vi "AlliGator Phasor Ratio Actions.vi"(0 "AlliGator Q Elements in":T6[](array[typedef]), 1 "VI in":refnum<vi>, 2 "Script in":bool, 5 "data value reference in":refnum<data-value>, 7 "AlliGator Q Event in":T7=enum."GUI:Idle", 9 "Data":variant, 11 "error in (no error)":errorcluster, 12 "AlliGator Ctrl Refnums":T8) -> (3 "Script out":bool, 4 "AlliGator Q Elements out":T6[](array[typedef]), 6 "Data Value Reference out":refnum<data-value>, 10 "[Notebook Message]":T1[](array[typedef]) {"Message Style"."Font Size" min=6.0 step=1.0}, 15 "error out":errorcluster)   [LabVIEW 2021, in "AlliGator Action Engine.lvlib"]
doc: "Processes AlliGator phasor ratio-related actions."
uses:
  AlliGator Action Engine.lvlib
  Internal Variables/AlliGator Internal Variables v2.ctl
  <vilib>/vision/Image Controls.llb/IMAQ Image.ctl
  Internal Variables/AlliGator Gate Image Set.ctl
  Files/AlliGator FLI Dataset Type.ctl
  Files/AlliGator Data Series Type.ctl
  Dual-Channel Datasets/AlliGator Dataset Channel.ctl
  Settings/AlliGator Gate Arithmetic.ctl
  Source Image/AlliGator Displayed Image.ctl
  Image/Named ROI Description.ctl
  Phasor Graph/AlliGator Decay Metadata v3.ctl
  Decay Analysis/Decay Preprocessing/AlliGator Decay Background Subtraction Info.ctl
  Decay Analysis/Decay Preprocessing/AlliGator Baseline Subtraction Method.ctl
  Graphs/XY Graph/XY Graph Plot Shift Parameters.ctl
  Graphs/XY Graph/XY Graph Plot Shift Method.ctl
  Decay Analysis/Decay Preprocessing/AlliGator Decay Extrapolation Parameters.ctl
  Phasor/Calibration Phasor (m, phi).ctl
  Phasor/Phasor Reference Series.ctl
  Phasor/Phasor Calibration Map v2.ctl
  Phasor/Phasor (g, s).ctl
  Phasor Graph/AlliGator Raw Phasor Plot Data v5.ctl
  Phasor/Phasor Standard Deviation Options.ctl
  Phasor Plot/AlliGator Phasor Multi-Harmonic Data.ctl
  Phasor/Phasor Harmonic Data.ctl
  Decay Fit Parameter Map/AlliGator Decay Fit Options & Parameters v3.ctl
  Fits/IRF(X)PSED/Decay Fit Options v3.ctl
  Fits/Decay Convolution/Decay Model.ctl
  Fits/Residual Type.ctl
  Fits/IRF(X)PSED/Fit Weights Type.ctl
  Fits/Non-linear Fitting Method v2.ctl
  Fits/Fit Calculation Method.ctl
  Fits/Non-linear Fitting Algorithm.ctl
  Decay Analysis/Decay Fit/AlliGator Decay Fit Parameter Constraints 2.ctl
  Fits/IRF(X)PSED/Decay Fit Parameters In List.ctl
  Fits/IRF(X)PSED/MLE Baseline Offset Type.ctl
  Decay Analysis/Decay Preprocessing/AlliGator Decay Preprocessing Parameters.ctl
  Fits/IRF(X)PSED/Decay Fit Parameters & Derived Quantities List v2.ctl
  Fits/IRF(X)PSED/Decay Fit Result Constraint.ctl
  Decay Fit Parameter Map/AlliGator Parameter Maps Data.ctl
  AlliGator Q Event.ctl
  GUI/AlliGator Ctrl Refnums.ctl
  GUI/AlliGator Other Ctrl Refnums.ctl
  GUI/AlliGator State Indicator.ctl
  GUI/AlliGator Main Window Tabs.ctl
  GUI/AlliGator Phasor Plot Ctrl Refnums.ctl
  GUI/AlliGator Phasor Graph Ctrl Refnums.ctl
  Phasor/Phasor Calibration Type.ctl
  GUI/AlliGator Dataset Ctrl Refnums.ctl
  GUI/AlliGator Registered Events Ctrl Refnums.ctl
  GUI/AlliGator Image Histogram Control Refnums.ctl
  Histograms/Linear Histogram Options.ctl
  Histograms/Histogram Bin Option.ctl
  Histograms/Histogram Bin Position.ctl
  Decay Fit Parameter Map/AlliGator Decay Fit Map Control Refnums.ctl
  Parameter Map/AlliGator Parameter Map Control Refnums.ctl
  AlliGator Q Element.ctl
  Notebook/Notebook Message Object.ctl
  Rich Text Box/Text Formatting.ctl
  Rich Text Box/Text Colors.ctl
  Rich Text Box/Text Style.ctl
  Rich Text Box/Text Alignment.ctl
  Rich Text Box/Text Format List.ctl
  Phasor Ratio/AlliGator Phasor Ratio at Mouse Location Data.ctl
  Graphs/XY Graph/XY Graph Mouse Click Event Data.ctl
  Graphs/XY Graph/XY Graph Refnum.ctl
  <vilib>/Utility/miscctls.llb/LVPoint32TypeDef.ctl
  Phasor Ratio/AlliGator Phasor Reference Data.ctl
  Alligator Elements Order in Action Stack.ctl
  AlliGator State Indicators List.ctl
  Globals, Variables, Constants/AlliGator Variables List.ctl
  Variant/Variant to Data/Variant to I32.vi
  Graphs/Get Plot at Mouse Click (XY Graph)/Get Plot at Mouse Click [AAC].vi
  Variant/Variant to Data/Variant to Boolean.vi
  Variant/Variant to Data/Variant to Path.vi
  AlliGator Add Single Action to Stack.vi
  Variant/Variant to Data/Variant to DBL.vi
  Variant/Variant to Data/Variant to Data.lvlib
  GUI/GUI.lvlib
  Source Image/AlliGator Source Image.lvlib
  Phasor Graph/AlliGator Phasor Graph.lvlib
  Phasor Ratio/AlliGator Phasor Ratio.lvlib
  Internal Variables/AlliGator Internal Variables.lvlib
  Graphs/XY Graph/XY Graph Add-Ons.lvlib
  Graphs/Graphs.lvlib
  Globals, Variables, Constants/AlliGator Globals, Variables & Constants.lvlib
  GUI/AlliGator GUI.lvlib
  Settings/AlliGator Settings.lvlib
  Phasor Calibration/AlliGator Phasor Calibration.lvlib
  Notebook/Notebook.lvlib
  Phasor/Phasor.lvlib
  Image/Image.lvlib
  Decay Analysis/Decay Preprocessing/AlliGator Decay Preprocessing.lvlib
  Files/AlliGator Files.lvlib
  Phasor Plot/AlliGator Phasor Plot.lvlib
  Fits/Fits.lvlib
  Decay Analysis/Decay Fit/AlliGator Decay Fit.lvlib
  Decay Fit Parameter Map/AlliGator Decay Fit Parameter Map.lvlib
  Rich Text Box/Rich Text Box.lvlib
  Dual-Channel Datasets/AlliGator Dual-Channel Datasets.lvlib
  Histograms/Histogram Window.lvlib
  Parameter Map/AlliGator Parameter Map.lvlib
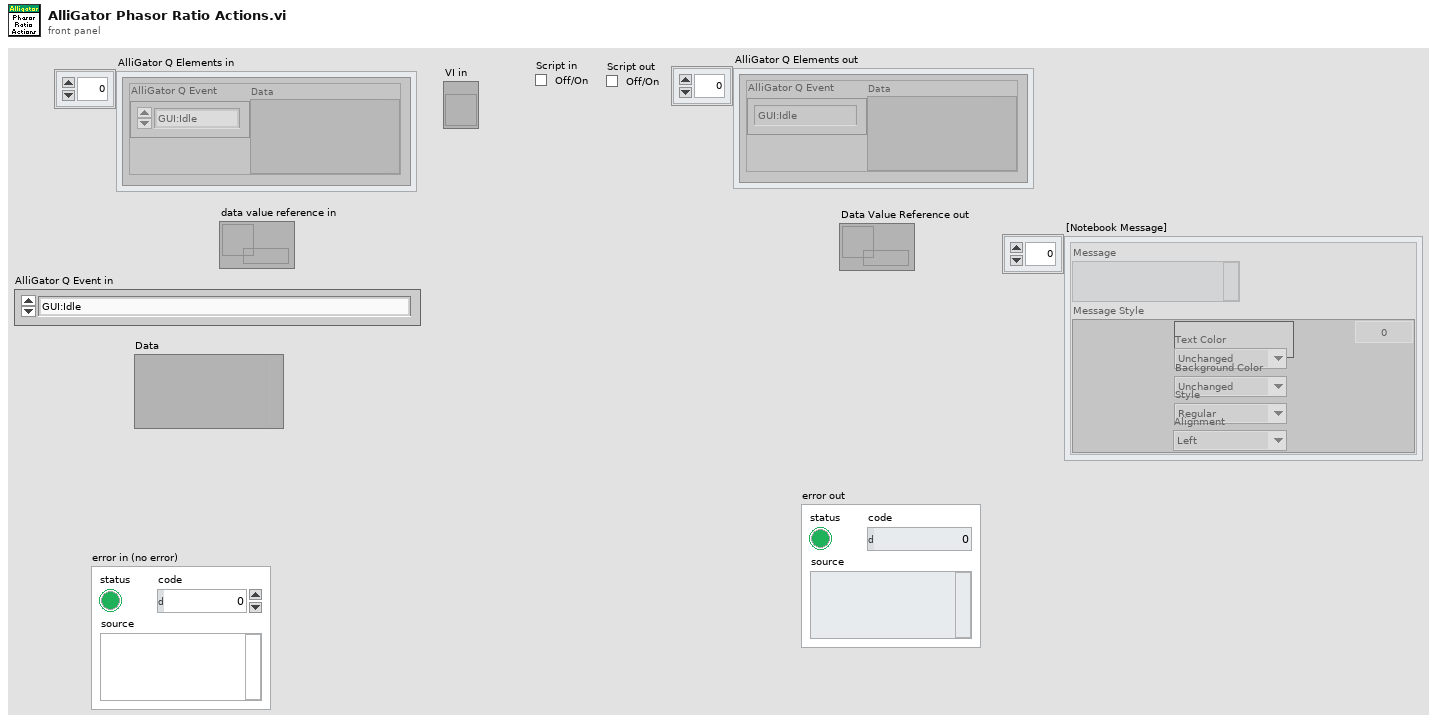
[diagram p1: front panel]
types:
  T1 = typedef "Notebook.lvlib/Notebook Message Object.ctl" = cluster{"Message":string, "Message Style":T2}
  T2 = typedef "Rich Text Box.lvlib/Text Formatting.ctl" = cluster{"Font":string, "Text Color":T3, "Background Color":T3, "Style":T4, "Font Size":dbl, "Alignment":T5}
  T3 = typedef "Rich Text Box.lvlib/Text Colors.ctl" = enum16{"Unchanged", "Black", "Blue", "Cyan", "Maroon", "Gray", "Violet", "Green", "Light Green", "Orange", "Yellow", "Magenta", "Red", "White"}
  T4 = typedef "Rich Text Box.lvlib/Text Style.ctl" = enum16{"Regular", "Bold", "Italic", "Underline", "Strikeout"}
  T5 = typedef "Rich Text Box.lvlib/Text Alignment.ctl" = enum16{"Left", "Right", "Center"}
  T6 = typedef "AlliGator Action Engine.lvlib/AlliGator Q Element.ctl" = cluster{"AlliGator Q Event":T7, "Data":variant}
  T7 = typedef "AlliGator Action Engine.lvlib/AlliGator Q Event.ctl" = enum16{"---- Files ----", "Files:Set Batch Export Files To Save", "Files:Set Dataset Loading & Pre-processing Options", "Files:Check #Frames in Dataset", "Files:Increment Frame Index", "Files:Open Mask Image", "Files:Open White Light Image", "Files:Open Single Dataset", "Files:New Folder of Folders Selected", "Files:Load File (all Types)_Scriptable", "Files:Move Flattened Series to Folders Series", "Files:Select Folder", "Files:Load FLI Dataset", "Files:Load Swiss SPAD 1 Dataset", "Files:Load Swiss SPAD 2 Dataset", "Files:Load .sdt FLI Dataset", "Files:Load .ptu FLI Dataset", "Files:Load .bin FLI Dataset", "Files:Load Single Gate Image Folder", "Files:Load I/m/phi Dataset (deprecated)", "Files:Load Single Image", "Files:Subtract Background File", "Files:Export FLI Dataset", "Files:Load HDF5 FLI Dataset", "Files:Set Destination File Path", "Files:Save Mask Image", "Files:Batch Conversion", "Files:New Folder Selected", "Files:Close FLI Dataset", "Files:Close FLI Dataset Series", "Files:Close White Light Image", "Files:Close Mask Image", "---- FLI Dataset ----", "FLI Dataset:Channel Arithmetic", "FLI Dataset:Export Average Lifetime Map as ASCII", "FLI Dataset:Export User-Defined Quantity Map as ASCII", "FLI Dataset:Python Function FLI Dataset Event", "FLI Dataset:ROI Analysis", "FLI Dataset:Tilted Logistic Square Gated IRF Characteristics Map", "FLI Dataset:Logistic Square Gated IRF Characteristics Map", "FLI Dataset:Square Gated IRF Characteristics Map", "FLI Dataset:Multi-ROI Single-Pixel Phasor Analysis", "FLI Dataset:Multi-ROI Single-Pixel NLSF Analysis", "FLI Dataset:All ROIs IRF Extraction", "FLI Dataset:All ROIs Decay Fit Non-Interactive (Fast + Individual IRF)", "FLI Dataset:All ROIs Phasor Analysis", "FLI Dataset:All ROIs Decay Fit", "FLI Dataset:Fluorescence Decay Statistics", "FLI Dataset:Update Decay Statistics Graph", "FLI Dataset:Get Decay from ROI", "FLI Dataset:All ROIs Average Lifetimes", "FLI Dataset:Save/Load Local IRFs", "FLI Dataset:Clear Local IRFs", "FLI Dataset:Phasor Calibration Maps (# Gates Series) Script", "FLI Dataset:Calibrated Phasor Map Series", "---- FLI Dataset Series ----", "FLI Dataset Series:Sum All Datasets in Series", "FLI Dataset Series:Add Dataset to Accumulated Dataset", "FLI Dataset Series:Display Accumulated Dataset", "FLI Dataset Series:Clear Dataset Series Sum", "FLI Dataset Series:Time-Series Analysis (NLSF)", "FLI Dataset Series:Time-Series Analysis (Phasor)", "---- Image ----", "Image:Update Image Profile Plots", "Image:Image Histogram Cursor Move", "Image:Image Histogram", "Image:Image Contrast", "Image:Set Image Histogram Cursor Move Flag", "Image:Clear Image Overlay", "Image:Use ROI as Search Area", "Image:Set ROI Diameter", "Image:Save Image Data as TIFF", "Image:Save Displayed Image with Overlay", "Image:Save Image Overlay Only", "Image:Save Image as Hot Pixel Mask", "Image:Change Source Image Color Palette", "Image:Copy Image to Clipboard", "Image:Source Image ROI Selection", "Image:Delete All ROIs", "Image:Delete All Unselected ROIs", "Image:Delete ROI", "Image:Merge All ROIs", "Image:Store ROI", "Image:Source Image ROI Storage", "Image:Export ROI Description to Notebook", "Image:Save ROI", "Image:Load ROI", "Image:Paste ROI Definition", "Image:Clear ROI", "Image:Identify ROIs in Mask Image", "Image:Create Complementary ROI", "Image:Create Contour ROI", "Image:Create ROI(s) from Pixels with Peak above Min_Scriptable", "Image:Create ROI(s) from Pixels with Intensity above Min_Scriptable", "Image:Compute ROI Statistics", "Image:Delete ROI(s) based on ROI Characteristics", "Image:Create ROI Grid", "Image:ROI to Individual Pixel ROIs", "Image:Python Function Source Image Event", "Image:Show Phasor Calibration Map ROI Centers", "Image:Convert ROI to Mask Image", "Image:Mouse Move", "Image:Mouse Up", "Image:Set Source Image Mouse Move Flag", "Image:Add Scale Bar Overlay", "Image:Delete Existing ROIs Option", "Image:Overlay ROI Median", "Image:Check Current ROI", "Image:Update True Pixel Value", "---- Decay ----", "Decay:Clear IRF/Reference Plot", "Decay:Add Decay to Graph", "Decay:Smoothen Plot", "Decay:Smoothen Plot Tail", "Decay:Average Selected Plots", "Decay:Extract IRF", "Decay:Optimal IRF Extraction", "Decay:Threshold IRF", "Decay:Fit to Model IRF", "Decay:Fit IRF to Square Gate", "Decay:Fit IRF to Logistic Square Gate", "Decay:Fit IRF to Tilted Logistic Square Gate", "Decay:Create Bounding Cursors Set", "Decay:Export Bounding Cursors Definition to Notebook", "Decay:Denoise Plot", "Decay:Compute Cumulative Function", "Decay:Use as Reference Decay", "Decay:Show Reference Decay/IRF", "Decay:Extrapolate Decay", "Decay:Create Head & Tail Bounding Cursors", "Decay:Store Cursor-defined Head & Tail Fractions", "Decay:Rebin Plot", "Decay:1-Normalize Decay", "Decay:[0-1]-Normalize Plot", "Decay:Straighten Decay", "Decay:Shift Decay", "Decay:Fold Decay", "Decay:Fit Decay", "Decay:Global Fit of Selected Decays", "Decay:Post Global Fit Script", "Decay:Add Global Fit Parameters to Graph", "Decay:Add Decay Parameter(s) to Plot (Graph)", "Decay:Export Decay to Phasor Graph", "Decay:Compute Average Lifetime", "Decay:Plot Convolution", "Decay:Graph Tip Strip Update", "---- Decay Statistics ----", "Decay Statistics:Tip Strip Update", "---- Intensity Time Trace ----", "Intensity Time Trace:Use File Timestamp", "Intensity Time Trace:Load Intensity Corrections File", "Intensity Time Trace:Clear Intensity Corrections File", "Intensity Time Trace:Tip Strip Update", "---- Phasor Plot ----", "Phasor Plot:Build Phasor Plot", "Phasor Plot:Change Phasor Plot Color Palette", "Phasor Plot:Adjust Phasor Plot Display Range", "Phasor Plot:Highlight Image ROI in Phasor Plot", "Phasor Plot:Save Phasor Plot Image with Overlay", "Phasor Plot:Export Complex Phasor Map", "Phasor Plot:Export Phasor Ratio Map", "Phasor Plot:Export Average Lifetime Map", "Phasor Plot:Compute Phase Lifetime Histogram", "Phasor Plot:Compute Phasor Ratio Histogram", "Phasor Plot:Compute Phase Lifetime vs Intensity Scatter Plot", "Phasor Plot:Weber 2-Component Decomposition", "Phasor Plot:Update Phasor Color Map Vertices", "Phasor Plot:Clear Phasor Overlay", "Phasor Plot:Use Segment Extremities as References", "Phasor Plot:Use UC/Segment Intersections as References", "Phasor Plot:Use UC/Principal Axis Intersections as References", "Phasor Plot:Use UC/Linear Fit Intersections as References", "Phasor Plot:Update Phasor Plot Reference", "Phasor Plot:Show Local Phasor Info in Phasor Plot", "Phasor Plot:Update Phasor Plot State", "Phasor Plot:Phasor Plot ROI Storage", "Phasor Plot:Phasor Plot ROI Selection", "Phasor Plot:Python Function Phasor Plot Event", "Phasor Plot:Overlay Phasor ROI, Ratio or Map in Source Image", "Phasor Plot:Compute Decay of Selected Phasors", "Phasor Plot:Phasor at Image Pixel", "Phasor Plot:Mouse Move", "Phasor Plot:Mouse Up", "Phasor Plot:Display Range Mouse Move", "Phasor Plot:Set Mouse Move Flag", "Phasor Plot:Update True Phasor Plot Value", "---- Phasor Graph ----", "Phasor Graph:Get Phasor Value", "Phasor Graph:Create New Phasor Plot Dialog", "Phasor Graph:Update Last Phasor Value", "Phasor Graph:Update Phasor (m, phi)", "Phasor Graph:Remove Single Phasor from Plot", "Phasor Graph:Add Single Phasor to Plot", "Phasor Graph:Remove Phasor Plot", "Phasor Graph:Remove Selected Phasor Plots", "Phasor Graph:Clear Phasor Data", "Phasor Graph:Clear Phasor Graph", "Phasor Graph:Cursor Move", "Phasor Graph:Draw Cursor Connecting Line", "Phasor Graph:Clear Cursor Connecting Line", "Phasor Graph:Find UC Intersection", "Phasor Graph:Use UC/Cursor-Defined Line Intersections", "Phasor Graph:Use Selected Plots Fitted Line/UC Intersections", "Phasor Graph:Use Selected Plots Principal Axis/UC Intersections", "Phasor Graph:Show Single Phasor", "Phasor Graph:Save Single Phasor Plot", "Phasor Graph:Save All Phasor Plots", "Phasor Graph:Load Phasor Plot(s)", "Phasor Graph:Phasor Multiplication", "Phasor Graph:Compute Average Phasor", "Phasor Graph:Compute Multiple Average Phasors (Selected Plots)", "Phasor Graph:Export Single Phasor Plot Phase Lifetimes", "Phasor Graph:Parameter 2 vs Parameter 1 Scatter Plot", "Phasor Graph:Use Cursor n Location", "Phasor Graph:Set Reference n to Current Phase Lifetime Value", "Phasor Graph:Set Reference n to Lifetime Value", "Phasor Graph:Set Cursor n Location", "Phasor Graph:Save Phasor Graph Image", "Phasor Graph:Update SEPL Plot", "Phasor Graph:Export Single Phasor Plot Data", "Phasor Graph:Export Selected Phasor Plots Data", "Phasor Graph:Python Function Phasor Graph Event", "Phasor Graph:Tip Strip Update", "---- Calibration ----", "Calibration:Set Calibration Type", "Calibration:Load/Save Phasor Calibration", "Calibration:Load/Save Phasor Calibration Series", "Calibration:Load/Save Phasor Calibration Map", "Calibration:Use as Calibration", "Calibration:Compute Optimal Calibration from Phasor References", "Calibration:Clear Phasor Calibration", "Calibration:Single Phasor Calibration Information", "Calibration:Use as Calibration Series", "Calibration:Use as Calibration Map", "Calibration:Clear Calibration Series", "Calibration:Phasor Calibration Series Information", "Calibration:Clear Calibration Map", "Calibration:Phasor Calibration Map Information", "Calibration:Apply Phasor Calibration", "Calibration:Update Single Plot Calibration", "Calibration:Update Multiple Plots Calibration", "Calibration:Clear Single Plot Calibration", "Calibration:Clear All Plots Calibrations", "Calibration:Clear Plot(s) Calibration(s)?", "---- Phasor Ratio ----", "Phasor Ratio:Clear Reference n", "Phasor Ratio:Toggle Selected Plot(s)  Lock to Reference 1", "Phasor Ratio:Use as Reference n", "Phasor Ratio:Send Reference n to Notebook", "Phasor Ratio:Toggle Selected Plot(s)  Lock to Reference 2", "Phasor Ratio:Compute Phasor Ratio at Mouse Location", "Phasor Ratio:Compute Phasor Plot's Average Phasor Ratio", "Phasor Ratio:Compute Time-Series Phasor Ratios", "Phasor Ratio:Fit Line to Phasor Ratio Plot", "Phasor Ratio:Save References", "Phasor Ratio:Load References", "Phasor Ratio:Update Phasor Reference 1", "Phasor Ratio:Update Phasor Reference 2", "Phasor Ratio:Move Cursor n to Reference n", "Phasor Ratio:Use as Phasor Reference 1 Lifetime", "Phasor Ratio:Use as Phasor Reference 2 Lifetime", "Phasor Ratio:Export Phasor Ratio Map as ASCII", "Phasor Ratio:Tip Strip Update", "---- Lifetime & Other Parameters Graph ----", "Lifetime:Compute Sliced Mean, SDV and CV Plots", "Lifetime:Plot Decay Shifts", "Lifetime:Plot Histogram", "---- Decay Fit Parameter Map ----", "Decay Fit Parameter Map:Export ROI NLSF Data as ASCII", "Decay Fit Parameter Map:Set Decay Fit Parameter Map Selection", "Decay Fit Parameter Map:Build Decay Fit Parameter Map", "Decay Fit Parameter Map:Change Decay Fit Parameter Map Color Palette", "Decay Fit Parameter Map:Export Decay Fit Parameter Map Data as ASCII", "Decay Fit Parameter Map:Export All Decay Fit Parameter Maps Data as ASCII", "Decay Fit Parameter Map:Selected Parameter Scatterplot", "Decay Fit Parameter Map:Parameter 2 vs Parameter 1 Scatterplot", "Decay Fit Parameter Map:Save Decay Fit Parameter Map Image", "Decay Fit Parameter Map:Save-Load IRFs & Fit Data", "Decay Fit Parameter Map:Update Local Decay Plots", "Decay Fit Parameter Map:Python Function Decay Fit Parameters Map Event", "Decay Fit Parameter Map:Overlay Decay Fit Parameter Map in Source Image", "Decay Fit Parameter Map:Selected Parameter vs Intensity Scatterplot", "Decay Fit Parameter Map:Mouse Up", "Decay Fit Parameter Map:Mouse Move", "Decay Fit Parameter Map:Display Range Mouse Move", "Decay Fit Parameter Map:Change Map Resolution", "Decay Fit Parameter Map:Variance Significance Maps", "Decay Fit Parameter Map:Fit Result Constraints Window", "---- Parameter Map ----", "Parameter Map:Export ROI Parameters Data as ASCII", "Parameter Map:Delete Parameter Map Set", "Parameter Map:Update Parameter List", "Parameter Map:Build Parameter Map", "Parameter Map:Change Parameter Map Color Palette", "Parameter Map:Export Parameter Map Data as ASCII", "Parameter Map:Export All Parameter Maps Data as ASCII", "Parameter Map:Selected Parameter Scatterplot", "Parameter Map:Parameter 2 vs Parameter 1 Scatterplot", "Parameter Map:Selected Parameter vs Intensity Scatterplot", "Parameter Map:Save Parameter Map Image", "Parameter Map:Save-Load IRFs & Parameter Maps (TODO)", "Parameter Map:Set Parameter Map Selection", "Parameter Map:Python Function Parameter Map Event", "Parameter Map:Overlay Parameter Map in Source Image", "Parameter Map:Update Local Decay Plots", "Parameter Map:Mouse Up", "Parameter Map:Mouse Move", "Parameter Map:Display Range Mouse Move", "---- Generic Graph ----", "Generic Graph:Generic XY Graph Event", "Generic Graph:Python Function XY Graph Event", "Generic Graph:New Plot", "Generic Graph:Save Plot", "Generic Graph:XY Plot Histogram", "Generic Graph:Set XY Graph Plot Name", "Generic Graph:Set Last Cursor Style", "Generic Graph:Tip Strip Update", "---- GUI ----", "GUI:Start Script", "GUI:Type of Displayed Image Changed", "GUI:Gate Image Slide Changed", "GUI:Show Busy Icon", "GUI:Show Busy Icon & Abort Button", "GUI:Hide Busy Icon", "GUI:Hide Busy Icon & Abort Button", "GUI:Abort", "GUI:End Script", "GUI:Start Timing", "GUI:End Timing", "GUI:Set State Indicator", "GUI:Send Parameters JSON Strings to Clipboard", "GUI:Set Gate Step", "GUI:Idle", "GUI:Initialization", "GUI:Quit", "GUI:Increment Dataset Index", "GUI:Set Dataset Index to -1", "GUI:Time Series Slider Moved", "GUI:Time Series Slider Changed", "GUI:Toggle Playback or Loop", "GUI:Playback Script", "GUI:Set Phasor Frequency", "GUI:Open Window", "GUI:Start Test Script", "GUI:End Test Script", "DEBUG"}
  T8 = typedef "AlliGator GUI.lvlib/AlliGator Ctrl Refnums.ctl" = cluster{"Other AlliGator Ctrl Refnums":T9, "Phasor Plot Ctrl Refnums":T10, "Phasor Graph Ctrl Refnums":T11, "Dataset Control Refnums":T12, "Registered Events Ctrl Refnums":T13, "Image Histogram Ctrl Refnums":T14, "Decay Fit Map Ctrl Refnums":T15, "Parameter Map Ctrl Refnums":T16}
  T9 = typedef "AlliGator GUI.lvlib/AlliGator Other Ctrl Refnums.ctl" = cluster{"State Indicators":refnum<vi>, " Progress Bar":refnum<vi>, "Decay Graph Active":refnum<vi>, "Decay Statistics Bin":refnum<vi>, "Time Step":refnum<vi>, "Use File Timestamp":refnum<vi>, "Tab Control":refnum<vi>, "CPU":refnum<vi>, "Abort Fit":refnum<vi>, "Dataset File/Folder Path":refnum<vi>, "Abort ROI Creation":refnum<vi>, "Event LED":refnum<vi>, "Dataset File/Folder Path 2":refnum<vi>, "Dataset File/Folder Path 3":refnum<vi>, "Dataset File/Folder Path 4":refnum<vi>, "Dataset File/Folder Path 5":refnum<vi>, "Dataset File/Folder Path 6":refnum<vi>, "Dataset File/Folder Path 7":refnum<vi>, "Dataset File/Folder Path 8":refnum<vi>, "Dataset File/Folder Path 9":refnum<vi>, "Dataset File/Folder Path 10":refnum<vi>, "Dataset File/Folder Path 11":refnum<vi>}
  T10 = typedef "AlliGator GUI.lvlib/AlliGator Phasor Plot Ctrl Refnums.ctl" = cluster{"Phasor Ratio":refnum<vi>, "Modulus Lifetime":refnum<vi>, "Phasor at cursor (m, phi)":refnum<vi>, "Phase Lifetime":refnum<vi>, "Phasor at cursor (g, s)":refnum<vi>, "Phasor Plor Average Lifetime":refnum<vi>, "Phasor Plot Active":refnum<vi>, "Save Phasor Plot":refnum<vi>, "Image Overlay Color":refnum<vi>, "Phasor Plot Color Scale":refnum<vi>, "Reference 1 Button":refnum<vi>, "Reference 2 Button":refnum<vi>, "True Phasor Plot Value":refnum<vi>}
  T11 = typedef "AlliGator GUI.lvlib/AlliGator Phasor Graph Ctrl Refnums.ctl" = cluster{"Phasor Ratio":refnum<vi>, "Modulus Lifetime":refnum<vi>, "Phasor at cursor (m, phi)":refnum<vi>, "Phase Lifetime":refnum<vi>, "Phasor at cursor (g, s)":refnum<vi>, "Phasor Graph Average Lifetime":refnum<vi>, "Phasor Graph Active":refnum<vi>, "Save Phasor Graph":refnum<vi>, "Phasor Frame Slide":refnum<vi>, "Single Step Phasor":refnum<vi>, "Calibration Type":refnum<vi>, "Show Line":refnum<vi>, "Phase Lifetime 1":refnum<vi>, "Phase Lifetime 2":refnum<vi>, "Phasor Graph Frequency":refnum<vi>, "Phasor Reference 1 Control":refnum<vi>, "Phasor Reference 2 Control":refnum<vi>, "Calibration Lifetime":refnum<vi>, "Phase Lifetime SDV":refnum<vi>, "Average Lifetime SDV":refnum<vi>, "Phasor Ratio SDV":refnum<vi>, "Modulus Lifetime SDV":refnum<vi>}
  T12 = typedef "AlliGator GUI.lvlib/AlliGator Dataset Ctrl Refnums.ctl" = cluster{"Current Data":refnum<vi>, "Gate Image Slide":refnum<vi>, "Time Point Slide":refnum<vi>, "Current Time Stamp":refnum<vi>, "Save Image":refnum<vi>, "Displayed Image":refnum<vi>, "Overlay Mode":refnum<vi>, "Phasor Overlay Color":refnum<vi>, "Image Color Scale":refnum<vi>, "Use ROI as Search Area":refnum<vi>, "Source Image ROI Color":refnum<vi>, "True Pixel Value":refnum<vi>}
  T13 = typedef "AlliGator GUI.lvlib/AlliGator Registered Events Ctrl Refnums.ctl" = cluster{"Time Point Slider":refnum<vi>, "Phasor Plot Display Range":refnum<vi>, "Decay Graph":refnum<vi>, "Decay Statistics Graph":refnum<vi>, "Intensity Time Trace":refnum<vi>, "Phasor Graph":refnum<vi>, "Phasor Ratio Graph":refnum<vi>, "Lifetime Graph":refnum<vi>, "Phasor Plot Display":refnum<vi>, "Source Image Display":refnum<vi>, "Decay Fit Parameter Map Display Range":refnum<vi>, "Decay Fit Parameter Map Display":refnum<vi>, "Parameter Map Display Range":refnum<vi>, "Parameter Map Display":refnum<vi>, "Phasor Plot Display Range":refnum<vi>}
  T14 = typedef "AlliGator GUI.lvlib/AlliGator Image Histogram Control Refnums.ctl" = cluster{"Image Histogram":refnum<vi>, "Image Histogram Options":refnum<vi>, "Image Histogram Active":refnum<vi>, "Image Histogram Upper Percentile":refnum<vi>, "Image Histogram Lower Percentile":refnum<vi>, "Auto-Adjust Contrast":refnum<vi>}
  T15 = typedef "AlliGator Decay Fit Parameter Map.lvlib/AlliGator Decay Fit Map Control Refnums.ctl" = cluster{"Decay Fit Parameter Map Color Scale":refnum<vi>, "Decay Fit Parameter":refnum<vi>, "Max Parameter":refnum<vi>, "Min Parameter":refnum<vi>, "Decay Fit Parameter Map Display":refnum<vi>, "Decay Fit Parameter Map Display Range":refnum<vi>, "Decay Parameter Map X":refnum<vi>, "Decay Parameter Map Y":refnum<vi>, "Decay Parameter Map Value":refnum<vi>}
  T16 = typedef "AlliGator Parameter Map.lvlib/AlliGator Parameter Map Control Refnums.ctl" = cluster{"Parameter Map Color Scale":refnum<vi>, "Map Parameter":refnum<vi>, "Max Parameter":refnum<vi>, "Min Parameter":refnum<vi>, "Parameter Map Display":refnum<vi>, "Parameter Map Display Range":refnum<vi>, "Parameter Map Set":refnum<vi>, "Parameter Map X":refnum<vi>, "Parameter Map Y":refnum<vi>, "Parameter Map Value":refnum<vi>}
  T17 = typedef "Notebook.lvlib/Text Format List.ctl" = enum16{"Message", "Result", "Error", "Setting", "Verbose", "Warning"}
  T18 = typedef "AlliGator Phasor Ratio.lvlib/AlliGator Phasor Ratio at Mouse Location Data.ctl" = cluster{"Mouse Click Event Data":T19, "Interactive?":bool}
  T19 = typedef "XY Graph Add-Ons.lvlib/XY Graph Mouse Click Event Data.ctl" = cluster{"Multiplot XY Graph":T20, "Mouse Coordinates":T21}
  T20 = typedef "XY Graph Add-Ons.lvlib/XY Graph Refnum.ctl" = refnum<vi>
  T21 = typedef "LVPoint32TypeDef.ctl" = cluster{"Horizontal":i32, "Vertical":i32}
  T22 = typedef "AlliGator Phasor Ratio.lvlib/AlliGator Phasor Reference Data.ctl" = cluster{"Data Type":string, "Data":variant}
  T23 = typedef "AlliGator Action Engine.lvlib/Alligator Elements Order in Action Stack.ctl" = enum16{"Enqueue 2 AFTER 1", "Enqueue 2 BEFORE 1"}
  T24 = typedef "AlliGator Globals, Variables & Constants.lvlib/AlliGator Variables List.ctl" = enum16{"---- GUI ----", "GUI:Initialization Status", "GUI:State Indicators Refnum", "GUI:Original AlliGator Menu Items", "GUI:Current Action Loop State", "GUI:Script in progress", "GUI:Playback", "GUI:Loop Playback", "GUI:Search ROI Used", "GUI:Search ROI", "Decay Graph Max Legend Size", "Intensity Graph Max Legend Size", "Decay Statistics Graph Max Legend Size", "Phasor Graph Max Legend Size", "Phasor Ratio Graph Max Legend Size", "Lifetime Graph Max Legend Size", "---- Files ----", "Files:Export Dataset Frames as Individual Files", "Files:Show Batch Export Help Balloons", "Files:Frames in Dataset", "Files:ptu File Frame Start Indices", "Files:Current Frame in Dataset", "Files:Current Frame Timestamp", "Files:Dataset Loaded", "Files:Dataset Metadata", "Files:Dataset Channel", "Files:Dataset Data Description", "Files:Background Dataset Metadata", "Files:Background Dataset Channel", "Files:Background Dataset Data Description", "Files:Background File Subtraction", "Files:Background File Path", "Files:Background File Pile-up Correction", "Files:Background File Pixel Well Capacity", "Files:Background File Scaling Factor", "Files:Current Dataset Load Settings", "Files:Dataset Path", "Files:ICCD-specific Information", "Files:Macrotime Gate Separation", "------ Python Plugins ------", "Python Plugins:Information", "Python Plugins:Python Session", "Python Plugins:Valid Python Session?", "---- Source Image ----", "Source Image:ROIs", "Source Image:Current ROI", "Source Image:ROI Event Refnum", "X_Source Image:Display Range", "X_Source Image:Palette Information", "X_Source Image:Type of Displayed Image", "X_Time Gate Slider", "Source Image:Palette List", "Source Image:Scale", "Source Image:ROI Overlay Color", "Source Image:Overlay to Erase", "Source Image:Is Displayed Image Accumulated", "Source Image:White Light Image Modified", "Source Image:Mask Image Modified", "---- Image Profile Window ----", "Image Profile:Window Event Refnum", "Image Profile:IntensityType", "Image Profile:Intensity Average Type", "Image Profile:Intensity-weighted SDV", "Image Profile:Box Profile Type", "Image Profile:Window Open", "Image Profile:Plotted Fit Parameter", "------ Phasor Graph -------", "Phasor Graph:Show Line", "---- Phasor Plot ---", "Phasor Plot:Parameters Changed", "Phasor Plot:FLI Dataset Modified since last Calculation", "Phasor Harmonics Data", "Selected Phasor Harmonics", "Phasor Harmonic Manager Event Refnum", "Phasor Plot:ROIs", "Phasor Plot:Current ROI", "Phasor Plot:ROI Event Refnum", "Phasor Plot:Image Reference Points", "Phasor Plot:Computed", "Phasor Plot:Palette Information", "Phasor Plot:Palette List", "Phasor Plot:Phasor Ratio Palette Information", "Phasor Plot:Phasor Ratio Palette List", "Phasor Plot:Image Scale", "Phasor Plot:Image Overlay to Erase", "Phasor Plot:Image Elements to Update", "Phasor Plot:Current Calculation Parameters", "Phasor Plot:Current Calibration Options", "Phasor Plot:Reset Cumulated Phasor Plot", "Phasor Plot:Reference 1", "Phasor Plot:Lifetime Reference 1", "Phasor Plot:Reference 1 Frequency", "Phasor Plot:Reference 2", "Phasor Plot:Lifetime Reference 2", "Phasor Plot:Reference 2 Frequency", "---- Decay Analysis ----", "Number of Selected Decays to Fit", "LS Fit Results", "LAR Fit Results", "BS Fit Results", "Last Decay Max - Min", "Best Fit Parameters", "Best Fit Parameter Names", "Actual Size X", "Actual Size Y", "Binning X", "Binning Y", "Actual # Gates", "Dataset Number", "Gates to...", "Gates Skipped", "Gates to keep", "Gate Step", "Gate Separation", "Reversed Gates", "Pile-up Correction", "Pixel Well Capacity", "Background Subtracted", "Background Subtraction Method", "Background Definition Range", "Background File (deprecated)", "Number of Dataset Accumulated", "Array of Accumulated Dataset Paths", "Do Averaged Datasets", "Destination File Path", "Process Plot Target", "Use 1/D as Phasor Frequency", "---- Decay Fit Parameter Map -----", "Decay Fit Parameter Map:Palette Information", "Decay Fit Parameter Map:Palette List", "Decay Fit Parameter Map:X Resolution", "Decay Fit Parameter Map:Y Resolution", "Decay Fit Parameter Map:Use Decay Fit Result Constraints", "Decay Fit Parameter Map:Decay Fit Result Constraints", "Decay Fit Parameter Map:Decay Fit Result Constraints Applied", "---- Parameter Map ----", "Parameter Map:Palette Information", "Parameter Map:Palette List", "------- Local Decay Window ---------", "Local Decay Graph Window:Event Refnum", "Local Decay Graph Window:Use normalized IRF for convolution", "----- Miscellaneous ----", "Misc:Skippable Dialog Windows Status"}
  T25 = typedef "AlliGator Action Engine.lvlib/AlliGator State Indicators List.ctl" = enum16{"Phasor Calibration Defined", "Phasor Calibration Series Defined", "Phasor Calibration Map Defined", "Phasor Reference 1 Defined", "Phasor Reference 2 Defined", "Lifetime Reference 1 Defined", "Lifetime Reference 2 Defined", "Phasor Calibration Used", "Phasor Calibration Series Used", "Phasor Calibration Map Used", "Dataset Update Needed", "Phasor Plot Update Needed", "Reference/IRF Defined", "Individual IRFs Defined"}
  T26 = typedef "Phasor.lvlib/Phasor (g, s).ctl" = cluster{"g":dbl, "s":dbl}
  T27 = cluster{"Phasor Ratio Reference 1":T26, "Reference Lifetime 1":dbl[unit], "Phasor Ratio Reference 2":T26, "Reference Lifetime 2":dbl[unit]}
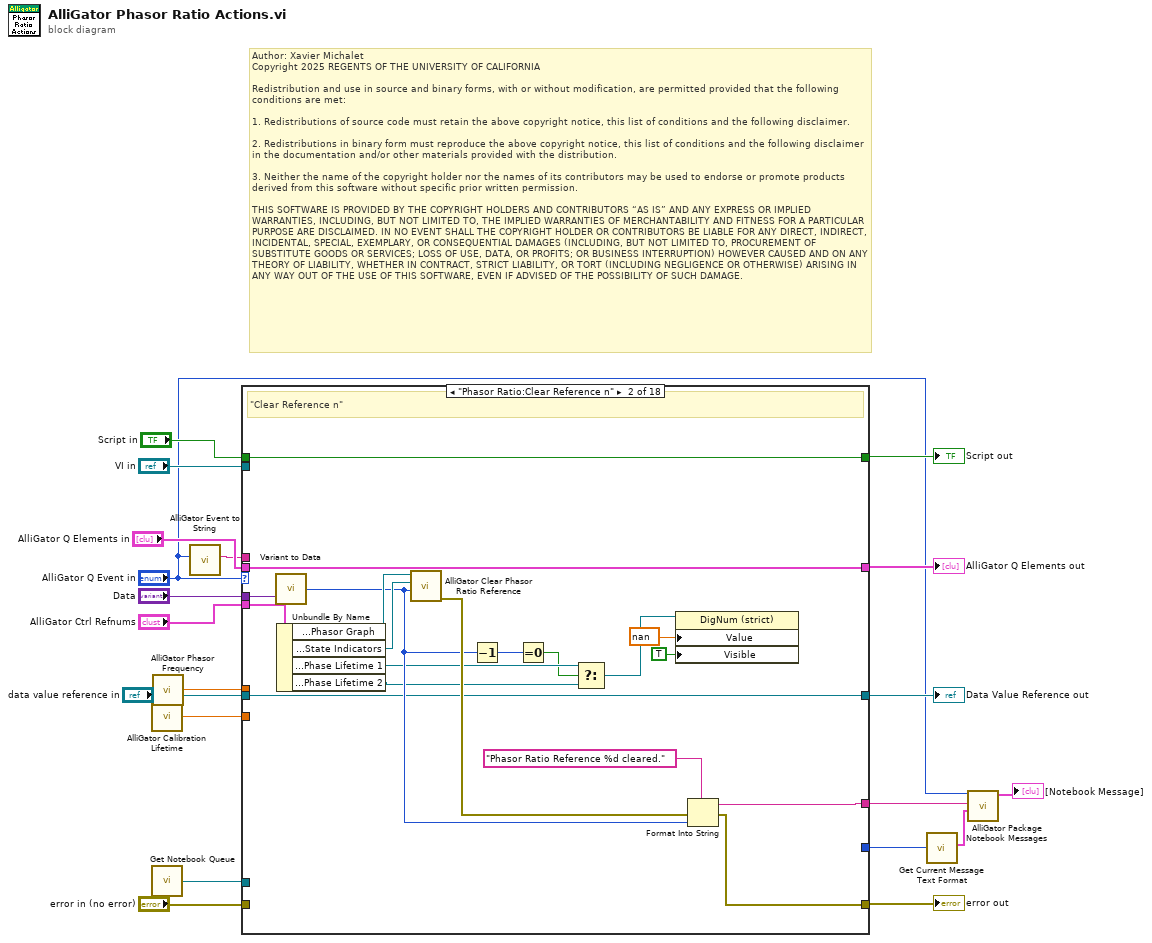
[diagram p0: block diagram]
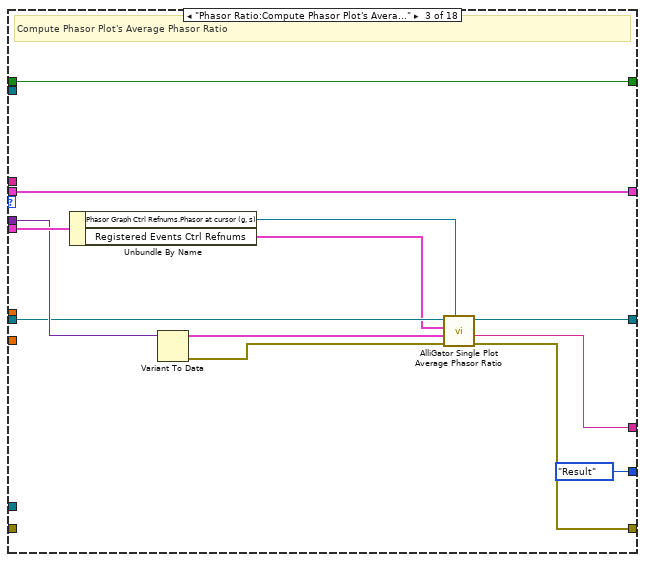
[diagram p3: hidden frame]
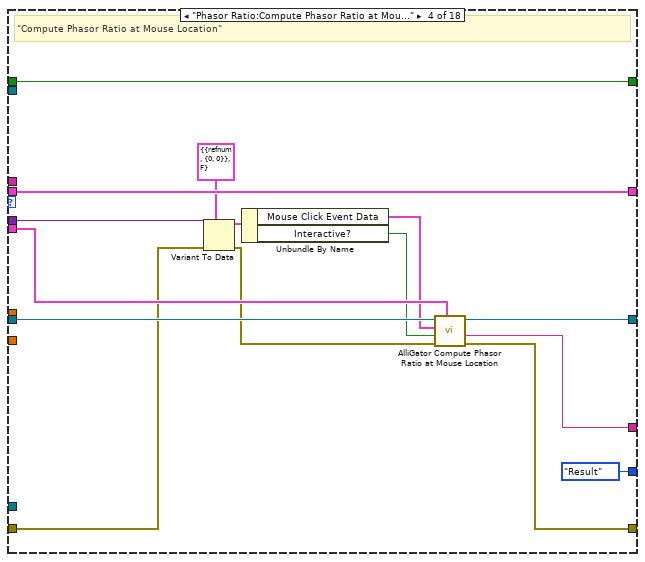
[diagram p4: hidden frame]
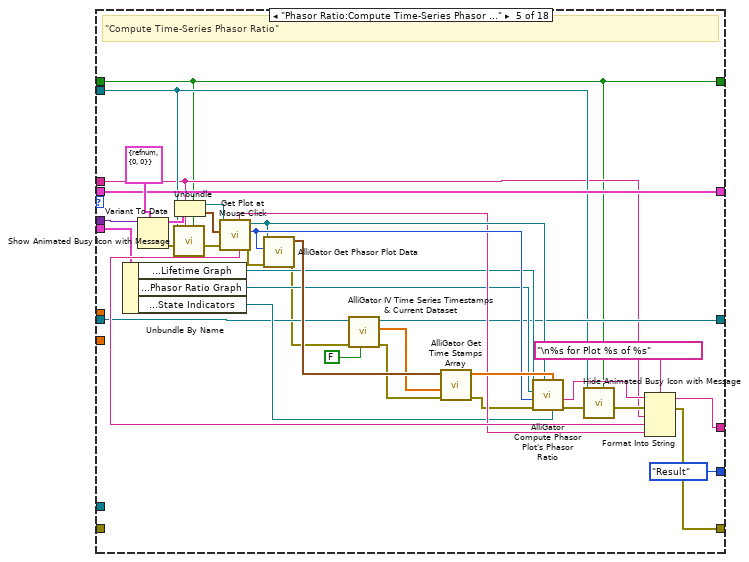
[diagram p5: hidden frame]
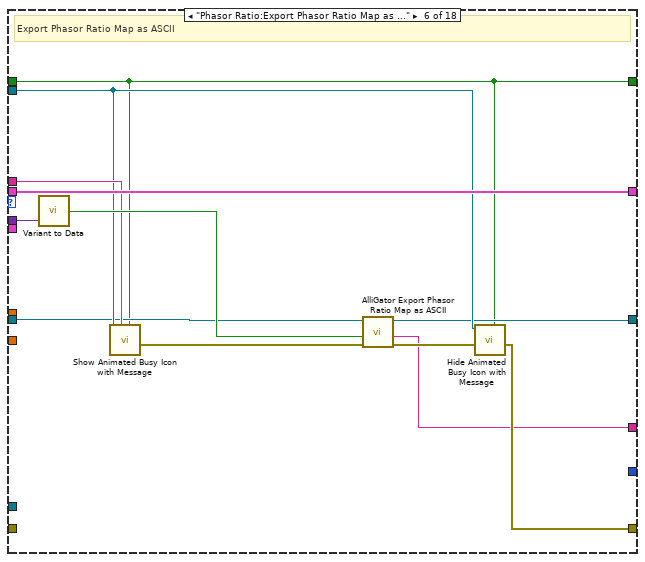
[diagram p6: hidden frame]
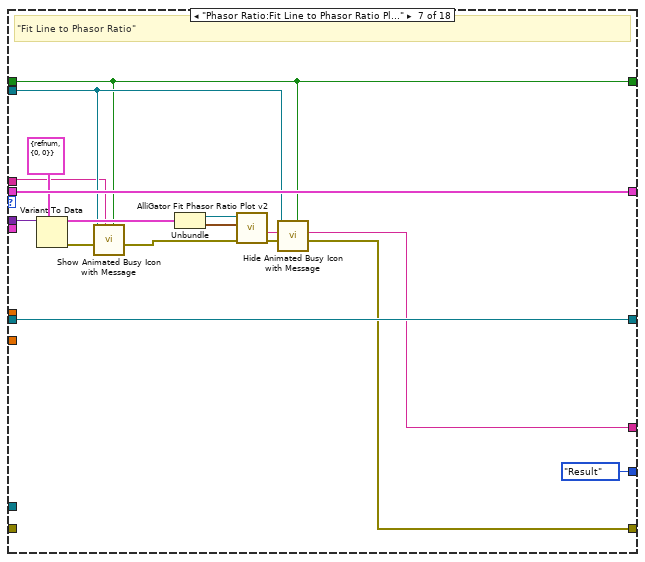
[diagram p7: hidden frame]
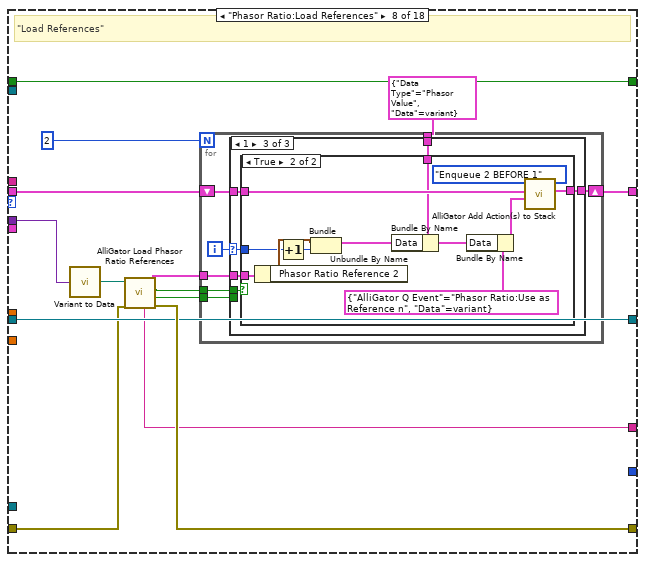
[diagram p8: hidden frame]
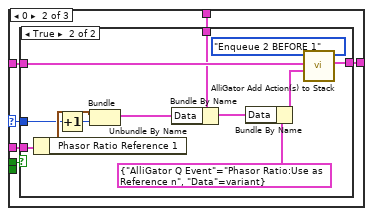
[diagram p10: hidden frame]
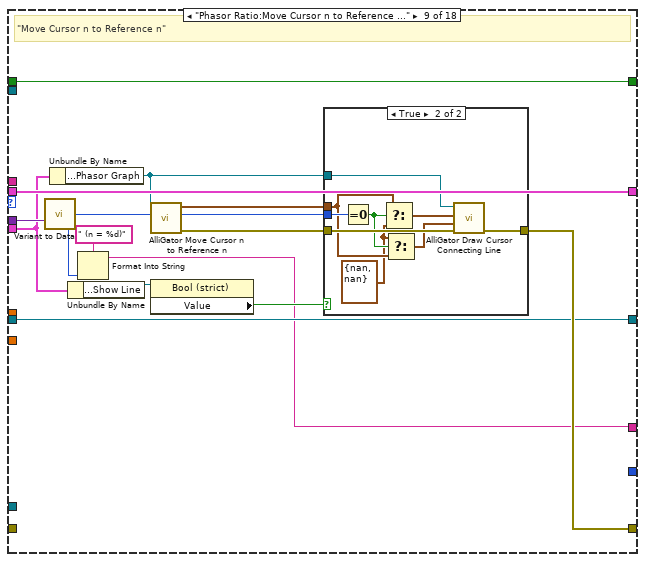
[diagram p13: hidden frame]
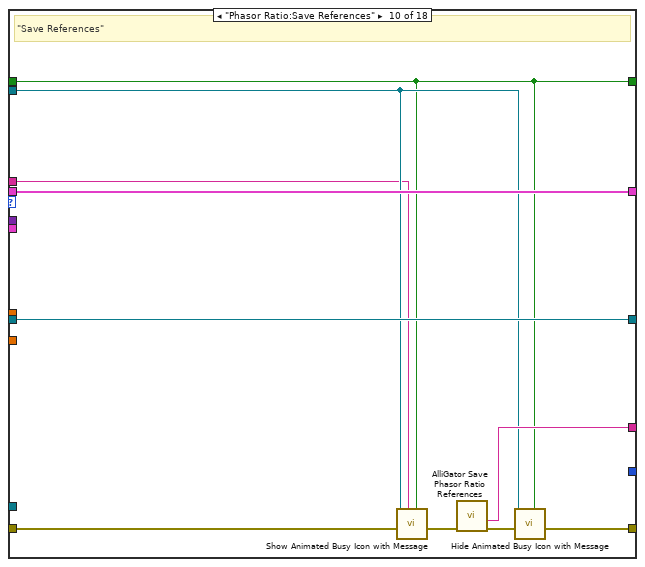
[diagram p15: hidden frame]
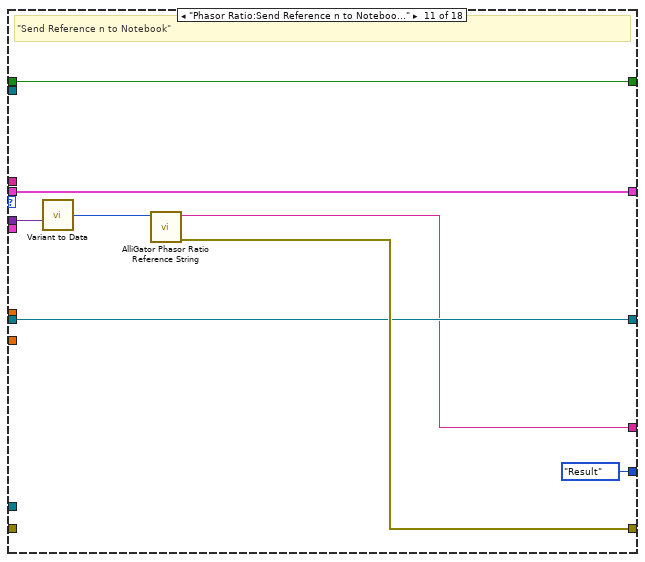
[diagram p16: hidden frame]
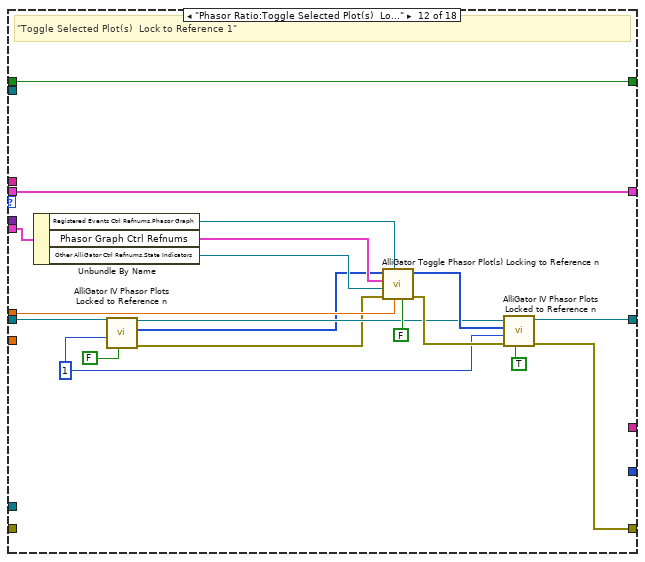
[diagram p17: hidden frame]
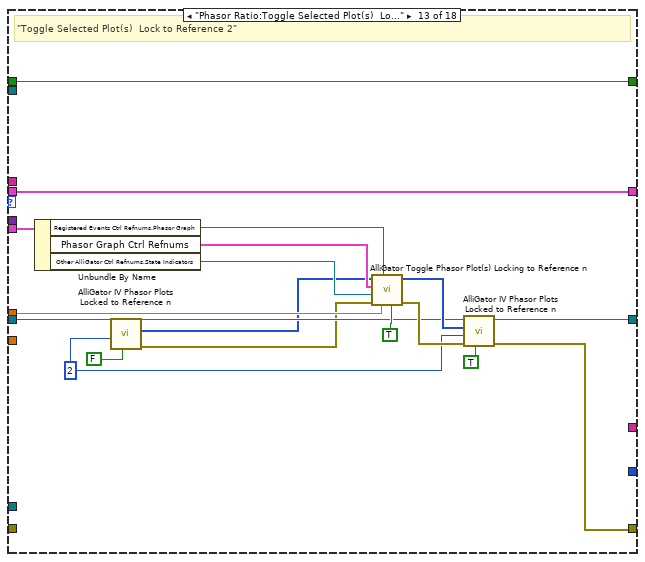
[diagram p18: hidden frame]
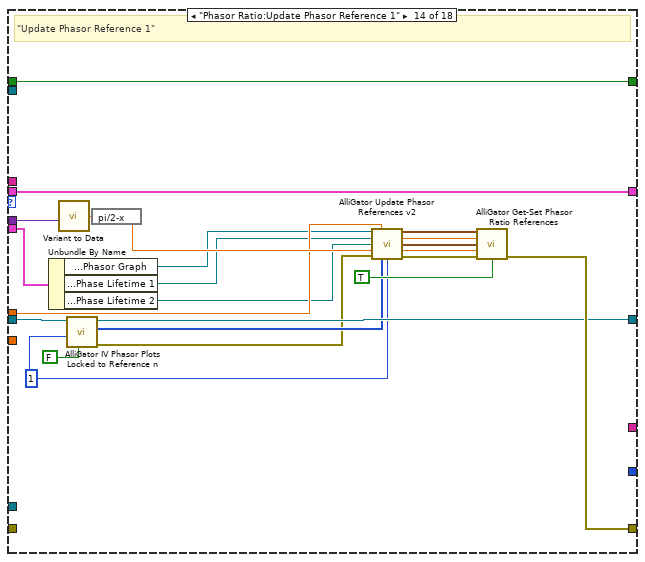
[diagram p19: hidden frame]
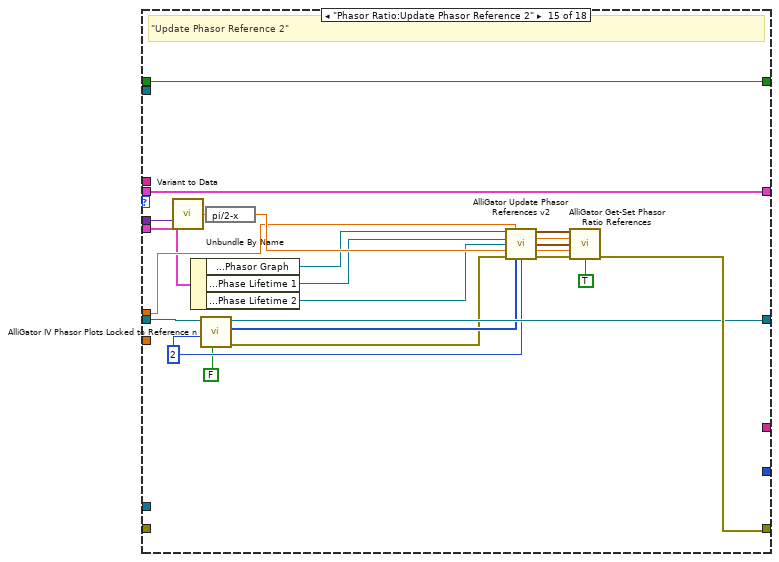
[diagram p20: hidden frame]
diagram:
  # "Author: Xavier Michalet\nCopyright 2025 REGENTS OF THE UNIVERSITY OF CALIFORNIA\n\nRedistribution and use in source and binary forms, with or without modification, are permitted provided that the following conditions are met:\n\n1. Redistributions of source code must retain the above copyright notice, this list of conditions and the following disclaimer.\n\n2. Redistributions in binary form must reproduce the above copyright notice, this list of conditions and the following disclaimer in the documentation and/or other materials provided with the distribution.\n\n3. Neither the name of the copyright holder nor the names of its contributors may be used to endorse or promote products derived from this software without specific prior written permission.\n\nTHIS SOFTWARE IS PROVIDED BY THE COPYRIGHT HOLDERS AND CONTRIBUTORS “AS IS” AND ANY EXPRESS OR IMPLIED WARRANTIES, INCLUDING, BUT NOT LIMITED TO, THE IMPLIED WARRANTIES OF MERCHANTABILITY AND FITNESS FOR A PARTICULAR PURPOSE ARE DISCLAIMED. IN NO EVENT SHALL THE COPYRIGHT HOLDER OR CONTRIBUTORS BE LIABLE FOR ANY DIRECT, INDIRECT, INCIDENTAL, SPECIAL, EXEMPLARY, OR CONSEQUENTIAL DAMAGES (INCLUDING, BUT NOT LIMITED TO, PROCUREMENT OF SUBSTITUTE GOODS OR SERVICES; LOSS OF USE, DATA, OR PROFITS; OR BUSINESS INTERRUPTION) HOWEVER CAUSED AND ON ANY THEORY OF LIABILITY, WHETHER IN CONTRACT, STRICT LIABILITY, OR TORT (INCLUDING NEGLIGENCE OR OTHERWISE) ARISING IN ANY WAY OUT OF THE USE OF THIS SOFTWARE, EVEN IF ADVISED OF THE POSSIBILITY OF SUCH DAMAGE."
  n1 = call "AlliGator Calibration Lifetime.vi"() -> ("Calibration Lifetime"=w18:dbl[unit])
  n2 = call "Get Notebook Queue.vi"() -> ("Notebook Queue"=w20:refnum<queue>)  [unwired: 9 in]
  n3 = call "AlliGator Phasor Frequency.vi"() -> ("Phasor Frequency"=w13:dbl[unit])
  n4 = call "AlliGator Event to String.vi"("AlliGator Q Event"="AlliGator Q Event in") -> ("String"=w7:string)  [unwired: 8 in]
  n5 = case shown="\"Phasor Ratio:Clear Reference n\"" "AlliGator Q Event in" {
    tunnel: "Data" -> [_ w43 w50 w65 w107 w118 w134 w138 w209 _ w235 _ _ w298 w320 _ _ w381]
    tunnel: "AlliGator Q Elements in" -> [w24 w38 w56 w71 w93 w119 w135 w145 w208 w229 w237 w256 w275 w276 w321 w335 w349 w380]
    tunnel: [w24 w38 w56 w71 w93 w119 w135 w143 w208 w229 w237 w256 w275 w276 w321 w335 w349 w380] -> w9
    tunnel: "VI in" -> [_ _ _ _ w75 w114 w123 _ _ w222 _ _ _ _ _ _ _ w368]
    tunnel: w20 -> [_ _ _ _ _ _ _ _ _ _ _ _ _ _ _ _ _ _]
    tunnel: w13 -> [_ _ _ _ _ _ _ _ _ _ _ w255 w272 w295 w317 _ _ _]
    tunnel: [w23 w40 w55 w69 w73 w108 w122 w142 w210 w220 w236 w254 w274 w294 w316 w333 w347 w354] -> w10
    tunnel: "Script in" -> [w23 w40 w55 w69 w73 w108 w122 w142 w210 w220 w236 w254 w274 w294 w316 w333 w347 w354]
    tunnel: w7 -> [_ _ _ _ w74 w115 w121 _ _ w221 _ _ _ _ _ _ _ w367]
    tunnel: "error in (no error)" -> [w22 _ _ w62 _ _ _ w136 _ w225 _ _ _ _ _ _ _ _]
    tunnel: [w22 w39 w54 w70 w91 w116 w124 w149 w206 w223 w233 w247 w266 w288 w310 w330 w344 w373] -> w16
    tunnel: "AlliGator Ctrl Refnums" -> [_ w36 w53 w64 w87 _ _ _ w200 _ _ w253 w273 w285 w307 w327 w341 w369]
    tunnel: w18 -> [_ _ _ _ _ _ _ _ _ _ _ _ _ _ _ w328 w342 _]
    tunnel: "data value reference in" -> [w21 w26 w46 w68 w84 w113 w127 w140 w197 w227 w232 w243 w262 w282 w304 w325 w339 w359]
    tunnel: [w21 w26 w47 w67 w85 w112 w127 w140 w197 w227 w232 w244 w265 w281 w303 w325 w339 w355] -> w6
    tunnel: [_ w25 w51 w66 w79 w109 w126 w139 w196 w226 w231 _ _ _ _ w324 _ w352] -> w5
    tunnel: [_ _ Text_Format_List."Result" ("Text Format") Text_Format_List."Result" ("Text Format") Text_Format_List."Result" ("Text Format") _ Text_Format_List."Result" ("Text Format") _ _ _ Text_Format_List."Result" ("Text Format") _ _ _ _ Text_Format_List."Result" ("Text Format") Text_Format_List."Result" ("Text Format") Text_Format_List."Result" ("Text Format")] -> w1
    frame "---- Phasor Ratio ----", Default {
      # "\"---- Phasor Ratio ----\""
    }
    frame "Phasor Ratio:Clear Reference n" {
      # "\"Clear Reference n\""
      n6 = call-poly "Variant to Data.vi"("Variant"=w43) -> ("Value"=w32:i32)  [unwired: 8 in]
      n7 = Unbundle By Name(w36) -> ("Registered Events Ctrl Refnums.Phasor Graph"=w34:refnum<vi>, "Other AlliGator Ctrl Refnums.State Indicators"=w35:refnum<vi>, "Phasor Graph Ctrl Refnums.Phase Lifetime 1"=w30:refnum<vi>, "Phasor Graph Ctrl Refnums.Phase Lifetime 2"=w28:refnum<vi>)
      n8 = call "AlliGator Clear Phasor Ratio Reference.vi"("Reference Number"=w32, "State Indicators Refnum"=w35, "Phasor Graph Refnum"=w34) -> ("Error Out"=w37:errorcluster)  [unwired: 8 in]
      n9 = Decrement(x=w32) -> (x-1=w31:i32)
      n10 = Equal To 0?(x=w31) -> (x = 0?=w29:bool)
      n11 = Select(t=w30, s=w29, f=w28) -> (s? t:f=w27:refnum<vi>)
      n12 = property class="DigNum (strict)"(reference=w27, "Value"=dbl[unit] nan ("Reference Lifetime 1"), "Visible"=TRUE) -> ()  [unwired: 1 in, 2 out]
      n13 = Format Into String(format string="Phasor Ratio Reference %d cleared." ("Message"), error in=w37, w32) -> (resulting string=w25:string, error out=w39:errorcluster)  [unwired: 1 in]
    }
    frame "Phasor Ratio:Compute Phasor Plot's Average Phasor Ratio" {
      # "Compute Phasor Plot's Average Phasor Ratio"
      n14 = Unbundle By Name(w53) -> ("Phasor Graph Ctrl Refnums.Phasor at cursor (g, s)"=w52:refnum<vi>, "Registered Events Ctrl Refnums"=w45:T13)
      n15 = Variant To Data(Variant=w50) -> (data=w49:T19, error out=w48:errorcluster)  [unwired: 2 in]
      n16 = call "AlliGator Single Plot Average Phasor Ratio.vi"("Current Phasor Ref"=w52, "Error In"=w48, "Mouse Click Event Data"=w49, "Registered Events Ctrl Refnums"=w45, "Data Value Reference in"=w46) -> ("Error Out"=w54:errorcluster, "Message"=w51:string, "Data Value Reference out"=w47:refnum<data-value>)  [unwired: 4 in]
    }
    frame "Phasor Ratio:Compute Phasor Ratio at Mouse Location" {
      # "\"Compute Phasor Ratio at Mouse Location\""
      n17 = Variant To Data(error in=w62, type=T18 {"Mouse Click Event Data"={"Multiplot XY Graph"=refnum, "Mouse Coordinates"={"Horizontal"=0, "Vertical"=0}}, "Interactive?"=FALSE} ("output cluster"), Variant=w65) -> (data=w61:T18, error out=w63:errorcluster)
      n18 = Unbundle By Name(w61) -> ("Mouse Click Event Data"=w60:T19, "Interactive?"=w59:bool)
      n19 = call "AlliGator Compute Phasor Ratio at Mouse Location.vi"("AlliGator Ctrl Refnums"=w64, "error in (no error)"=w63, "Interactive?"=w59, "Mouse Click Event Data"=w60, "Data Value Reference in"=w68) -> ("error out"=w70:errorcluster, "Message"=w66:string, "Data Value Reference out"=w67:refnum<data-value>)  [unwired: 4 in]
    }
    frame "Phasor Ratio:Compute Time-Series Phasor Ratios" {
      # "\"Compute Time-Series Phasor Ratio\""
      n20 = Unbundle By Name(w87) -> ("Registered Events Ctrl Refnums.Lifetime Graph"=w89:refnum<vi>, "Registered Events Ctrl Refnums.Phasor Ratio Graph"=w88:refnum<vi>, "Other AlliGator Ctrl Refnums.State Indicators"=w86:refnum<vi>)
      n21 = Variant To Data(type=T19 {"Multiplot XY Graph"=refnum, "Mouse Coordinates"={"Horizontal"=0, "Vertical"=0}} ("Mouse Click Event Data"), Variant=w107) -> (data=w103:T19, error out=w100:errorcluster)  [unwired: 1 in]
      n22 = call "Show Animated Busy Icon with Message.vi"("Already active? (F)"=w73, "Message"=w74, "Error In"=w100, "Target VI Refnum"=w75) -> ("Error Out"=w76:errorcluster)  [unwired: 7 in]
      n23 = Unbundle(w103) -> ("Multiplot XY Graph"=w102:T20, "Mouse Coordinates"=w101:T21)
      n24 = call-poly "Get Plot at Mouse Click.vi"("error in (no error)"=w76, "Mouse Click Coordinates"=w101, "XY Graph in"=w102) -> ("error out"=w99:errorcluster, "Plot at Coordinates"=w97:i32, "XY Graph out"=w96:T20, "Plot Name"=w94:string, "Graph Name"=w90:string)  [unwired: 2 in, 2 out]
      n25 = call "AlliGator Get Phasor Plot Data.vi"("error in (no error)"=w99, "Plot Idx (-1: last)"=w97, "Phasor Graph Refnum"=w96) -> ("error out"=w82:errorcluster, "Phasor Array"=w98:T26[])  [unwired: 5 in, 2 out]
      n26 = call "AlliGator IV Time Series Timestamps & Current Dataset.vi"("Get (F)/ Set"=FALSE ("Get (F)/ Set (T)"), "error in (no error)"=w82, "AlliGator IV DVR in"=w84) -> ("error out"=w81:errorcluster, "[Time-Series Timestamps]"=w83:dbl[], "AlliGator IV DVR out"=w85:refnum<data-value>)  [unwired: 5 in, 1 out]
      n27 = call "AlliGator Get Time Stamps Array.vi"("Error In"=w81, "Dataset Series Timestamps in"=w83, "Phasor Array"=w98) -> ("Error Out"=w77:errorcluster, "Dataset Series Timestamps out"=w105:dbl[])  [unwired: 7 in]
      n28 = call "AlliGator Compute Phasor Plot's Phasor Ratio.vi"("State Indicators Refnum"=w86, "Time Stamp Array"=w105, "Phasor Graph"=w96, "Error In"=w77, "Plot Idx"=w97, "Phasor Ratio Graph"=w88, "Lifetime Graph"=w89) -> ("Error Out"=w106:errorcluster, "Message"=w78:string)  [unwired: 3 in]
      n29 = call "Hide Animated Busy Icon with Message.vi"("Already active? (F)"=w73, "Error In"=w106, "Target VI reference"=w75) -> ("Error Out"=w92:errorcluster)  [unwired: 8 in]
      n30 = Format Into String(format string="\n%s for Plot %s of %s", initial string=w78, error in=w92, w74, w94, w90) -> (resulting string=w79:string, error out=w91:errorcluster)
    }
    frame "Phasor Ratio:Export Phasor Ratio Map as ASCII" {
      # "Export Phasor Ratio Map as ASCII"
      n31 = call-poly "Variant to Data.vi"("Variant"=w118) -> ("Value"=w117:bool)  [unwired: 8 in]
      n32 = call "Show Animated Busy Icon with Message.vi"("Already active? (F)"=w108, "Message"=w115, "Target VI Refnum"=w114) -> ("Error Out"=w111:errorcluster)  [unwired: 8 in]
      n33 = call "AlliGator Export Phasor Ratio Map as ASCII.vi"("error in (no error)"=w111, "Dialog?"=w117, "Data Value Reference in"=w113) -> ("error out"=w110:errorcluster, "Message"=w109:string, "Data Value Reference out"=w112:refnum<data-value>)  [unwired: 6 in]
      n34 = call "Hide Animated Busy Icon with Message.vi"("Already active? (F)"=w108, "Error In"=w110, "Target VI reference"=w114) -> ("Error Out"=w116:errorcluster)  [unwired: 8 in]
    }
    frame "Phasor Ratio:Fit Line to Phasor Ratio Plot" {
      # "\"Fit Line to Phasor Ratio\""
      n35 = Variant To Data(type=T19 {"Multiplot XY Graph"=refnum, "Mouse Coordinates"={"Horizontal"=0, "Vertical"=0}} ("Mouse Click Event Data"), Variant=w134) -> (data=w131:T19, error out=w132:errorcluster)  [unwired: 1 in]
      n36 = call "Show Animated Busy Icon with Message.vi"("Already active? (F)"=w122, "Message"=w121, "Error In"=w132, "Target VI Refnum"=w123) -> ("Error Out"=w125:errorcluster)  [unwired: 7 in]
      n37 = Unbundle(w131) -> ("Multiplot XY Graph"=w130:T20, "Mouse Coordinates"=w128:T21)
      n38 = call "AlliGator Fit Phasor Ratio Plot v2.vi"("Error In"=w125, "Mouse Coordinates"=w128, "Phasor Ratio Graph Ref"=w130) -> ("Error Out"=w129:errorcluster, "Message"=w126:string)  [unwired: 5 in, 2 out]
      n39 = call "Hide Animated Busy Icon with Message.vi"("Already active? (F)"=w122, "Error In"=w129, "Target VI reference"=w123) -> ("Error Out"=w124:errorcluster)  [unwired: 8 in]
    }
    frame "Phasor Ratio:Load References" {
      # "\"Load References\""
      n40 = call-poly "Variant to Data.vi"("Variant"=w138) -> ("Path"=w137:path)  [unwired: 8 in]
      n41 = call "AlliGator Load Phasor Ratio References.vi"("Error In"=w136, "Reference File Path (default: Dialog)"=w137) -> ("Error Out"=w149:errorcluster, "Reference 2 Loaded"=w144:bool, "Reference 1 Loaded"=w148:bool, "Phasor References"=w147:T27, "Message"=w139:string)  [unwired: 5 in]
      n42 = for {
        N: 2 -> [_]
        tunnel: w148 -> [w154]
        tunnel: w147 -> [w156]
        shift-right: [w152] -> w143
        shift-left: w145 -> [w153]
        tunnel: w144 -> [w151]
        tunnel: T22 {"Data Type"="Phasor Value", "Data"=variant} ("Phasor Reference Data") -> [w150]
        i -> [w155]
        n43 = case shown="1" w155 {
          selector: w155 -> [_ w159 w178]
          tunnel: w156 -> [_ w163 w182]
          tunnel: w154 -> [_ w162 w181]
          tunnel: w153 -> [w157 w161 w180]
          tunnel: [w157 w160 w179] -> w152
          tunnel: w151 -> [_ _ _]
          tunnel: w150 -> [_ w158 w177]
          frame -1, Default {
          }
          frame 0 {
            n44 = case shown="True" w162 {
              tunnel: w163 -> [_ w176]
              tunnel: w161 -> [w164 w175]
              tunnel: [w164 w174] -> w160
              tunnel: w159 -> [_ w169]
              tunnel: w158 -> [_ w167]
              frame False {
              }
              frame True {
                n45 = Unbundle By Name(w176) -> ("Phasor Ratio Reference 1"=w170:T26)
                n46 = Increment(x=w169) -> (x+1=w168:i32)
                n47 = Bundle("Phasor Ratio Reference 1"=w170, w168) -> (w165:cluster{"Phasor Ratio Reference 1":T26, i32})  [unwired: 1 in]
                n48 = Bundle By Name(cluster=w167, "Data"=w165) -> (w166:T22)
                n49 = Bundle By Name(cluster=T6 {"AlliGator Q Event"=enum."Phasor Ratio:Use as Reference n", "Data"=variant} ("Alligator Atomic Action"), "Data"=w166) -> (w171:T6)
                n50 = call-poly "AlliGator Add Action(s) to Stack.vi"("Elements Order in Action Stack (Default: 2 BEFORE 1)"=Alligator_Elements_Order_in_Action_Stack."Enqueue 2 BEFORE 1", "Alligator Atomic Action"=w171, "Alligator Queue Element 1"=w175) -> ("Alligator Queue Element 1 (+ 2)"=w174:T6[])  [unwired: 7 in, 1 out]
              }
            }
          }
          frame 1 {
            n51 = case shown="True" w181 {
              tunnel: w182 -> [_ w195]
              tunnel: w180 -> [w183 w194]
              tunnel: [w183 w193] -> w179
              tunnel: w178 -> [_ w188]
              tunnel: w177 -> [_ w186]
              frame False {
              }
              frame True {
                n52 = Unbundle By Name(w195) -> ("Phasor Ratio Reference 2"=w189:T26)
                n53 = Increment(x=w188) -> (x+1=w187:i32)
                n54 = Bundle("Phasor Ratio Reference 2"=w189, w187) -> (w184:cluster{"Phasor Ratio Reference 2":T26, i32})  [unwired: 1 in]
                n55 = Bundle By Name(cluster=w186, "Data"=w184) -> (w185:T22)
                n56 = Bundle By Name(cluster=T6 {"AlliGator Q Event"=enum."Phasor Ratio:Use as Reference n", "Data"=variant} ("Alligator Atomic Action"), "Data"=w185) -> (w190:T6)
                n57 = call-poly "AlliGator Add Action(s) to Stack.vi"("Elements Order in Action Stack (Default: 2 BEFORE 1)"=Alligator_Elements_Order_in_Action_Stack."Enqueue 2 BEFORE 1", "Alligator Atomic Action"=w190, "Alligator Queue Element 1"=w194) -> ("Alligator Queue Element 1 (+ 2)"=w193:T6[])  [unwired: 7 in, 1 out]
              }
            }
          }
        }
      }
    }
    frame "Phasor Ratio:Move Cursor n to Reference n" {
      # "\"Move Cursor n to Reference n\""
      n58 = call-poly "Variant to Data.vi"("Variant"=w209) -> ("Value"=w202:i32)  [unwired: 8 in]
      n59 = Unbundle By Name(w200) -> ("Registered Events Ctrl Refnums.Phasor Graph"=w205:refnum<vi>)
      n60 = Unbundle By Name(w200) -> ("Phasor Graph Ctrl Refnums.Show Line"=w199:refnum<vi>)
      n61 = Format Into String(format string=" (n = %d)", w202) -> (resulting string=w196:string)  [unwired: 2 in, 1 out]
      n62 = call "AlliGator Move Cursor n to Reference n.vi"("Reference n"=w202, "Phasor Graph Refnum"=w205) -> ("Error Out"=w207:errorcluster, "Reference Idx"=w203:i32, "Reference Phasor"=w204:T26)  [unwired: 7 in]
      n63 = property class="Bool (strict)"(reference=w199) -> ("Value"=w198:bool)  [unwired: 1 in, 2 out]
      n64 = case shown="True" w198 {
        tunnel: w205 -> [_ w219]
        tunnel: [_ w218] -> w206
        tunnel: w207 -> [_ w217]
        tunnel: w204 -> [_ w213]
        tunnel: w203 -> [_ w216]
        frame False {
        }
        frame True {
          w212 = cluster{"X":dbl, "Y":dbl} {"X"=nan, "Y"=nan} ("Reference 2")
          n65 = Equal To 0?(x=w216) -> (x = 0?=w214:bool)
          n66 = Select(t=w213, s=w214, f=w212) -> (s? t:f=w215:T26)
          n67 = Select(t=w212, s=w214, f=w213) -> (s? t:f=w211:T26)
          n68 = call "AlliGator Draw Cursor Connecting Line.vi"("Error In"=w217, "Reference 2"=w211, "Reference 1"=w215, "Phasor Graph Refnum"=w219) -> ("Error Out"=w218:errorcluster)  [unwired: 7 in]
        }
      }
    }
    frame "Phasor Ratio:Save References" {
      # "\"Save References\""
      n69 = call "Show Animated Busy Icon with Message.vi"("Already active? (F)"=w220, "Message"=w221, "Error In"=w225, "Target VI Refnum"=w222) -> ("Error Out"=w224:errorcluster)  [unwired: 7 in]
      n70 = call "AlliGator Save Phasor Ratio References.vi"("Error In"=w224) -> ("Error Out"=w228:errorcluster, "Message"=w226:string)  [unwired: 9 in]
      n71 = call "Hide Animated Busy Icon with Message.vi"("Already active? (F)"=w220, "Error In"=w228, "Target VI reference"=w222) -> ("Error Out"=w223:errorcluster)  [unwired: 8 in]
    }
    frame "Phasor Ratio:Send Reference n to Notebook" {
      # "\"Send Reference n to Notebook\""
      n72 = call-poly "Variant to Data.vi"("Variant"=w235) -> ("Value"=w234:i32)  [unwired: 8 in]
      n73 = call "AlliGator Phasor Ratio Reference String.vi"("Reference #"=w234) -> ("Error Out"=w233:errorcluster, "Message"=w231:string)  [unwired: 9 in]
    }
    frame "Phasor Ratio:Toggle Selected Plot(s)  Lock to Reference 1" {
      w240 = 1 ("Reference n")
      # "\"Toggle Selected Plot(s)  Lock to Reference 1\""
      n74 = Unbundle By Name(w253) -> ("Registered Events Ctrl Refnums.Phasor Graph"=w249:refnum<vi>, "Phasor Graph Ctrl Refnums"=w252:T11, "Other AlliGator Ctrl Refnums.State Indicators"=w251:refnum<vi>)
      n75 = call "AlliGator IV Phasor Plots Locked to Reference n.vi"("Get (F)/ Set (T)"=FALSE, "Reference n"=w240, "AlliGator IV DVR in"=w243) -> ("error out"=w238:errorcluster, "[Phasor Plot(s) locked to Ref n"=w241:i32[], "AlliGator IV DVR out"=w242:refnum<data-value>)  [unwired: 6 in]
      n76 = call "AlliGator Toggle Phasor Plot(s) Locking to Reference n.vi"("Ref 1(F)/Ref 2(T)"=FALSE, "Phasor Frequency"=w255, "Phasor Graph Refnum"=w249, "error in"=w238, "State Indicators"=w251, "Phasor Graph Ctrl Refnums"=w252, "[Phasor Plot(s) locked to Ref n] in"=w241) -> ("error out"=w248:errorcluster, "[Phasor Plot(s) locked to Ref n] out"=w246:i32[])  [unwired: 3 in]
      n77 = call "AlliGator IV Phasor Plots Locked to Reference n.vi"("Get (F)/ Set (T)"=TRUE, "error in (no error)"=w248, "Reference n"=w240, "[Phasor Plot(s) locked to Ref n"=w246, "AlliGator IV DVR in"=w242) -> ("error out"=w247:errorcluster, "AlliGator IV DVR out"=w244:refnum<data-value>)  [unwired: 4 in, 1 out]
    }
    frame "Phasor Ratio:Toggle Selected Plot(s)  Lock to Reference 2" {
      w258 = 2 ("Reference n")
      # "\"Toggle Selected Plot(s)  Lock to Reference 2\""
      n78 = Unbundle By Name(w273) -> ("Registered Events Ctrl Refnums.Phasor Graph"=w268:refnum<vi>, "Phasor Graph Ctrl Refnums"=w271:T11, "Other AlliGator Ctrl Refnums.State Indicators"=w270:refnum<vi>)
      n79 = call "AlliGator IV Phasor Plots Locked to Reference n.vi"("Get (F)/ Set (T)"=FALSE, "Reference n"=w258, "AlliGator IV DVR in"=w262) -> ("error out"=w260:errorcluster, "[Phasor Plot(s) locked to Ref n"=w259:i32[], "AlliGator IV DVR out"=w261:refnum<data-value>)  [unwired: 6 in]
      n80 = call "AlliGator Toggle Phasor Plot(s) Locking to Reference n.vi"("Ref 1(F)/Ref 2(T)"=TRUE, "Phasor Frequency"=w272, "Phasor Graph Refnum"=w268, "error in"=w260, "State Indicators"=w270, "Phasor Graph Ctrl Refnums"=w271, "[Phasor Plot(s) locked to Ref n] in"=w259) -> ("error out"=w267:errorcluster, "[Phasor Plot(s) locked to Ref n] out"=w264:i32[])  [unwired: 3 in]
      n81 = call "AlliGator IV Phasor Plots Locked to Reference n.vi"("Get (F)/ Set (T)"=TRUE, "error in (no error)"=w267, "Reference n"=w258, "[Phasor Plot(s) locked to Ref n"=w264, "AlliGator IV DVR in"=w261) -> ("error out"=w266:errorcluster, "AlliGator IV DVR out"=w265:refnum<data-value>)  [unwired: 4 in, 1 out]
    }
    frame "Phasor Ratio:Update Phasor Reference 1" {
      w277 = 1 ("Reference n")
      # "\"Update Phasor Reference 1\""
      n82 = Unbundle By Name(w285) -> ("Registered Events Ctrl Refnums.Phasor Graph"=w286:refnum<vi>, "Phasor Graph Ctrl Refnums.Phase Lifetime 1"=w284:refnum<vi>, "Phasor Graph Ctrl Refnums.Phase Lifetime 2"=w283:refnum<vi>)
      n83 = call-poly "Variant to Data.vi"("Variant"=w298) -> ("Value"=w297:dbl)  [unwired: 8 in]
      n84 = call "AlliGator IV Phasor Plots Locked to Reference n.vi"("Get (F)/ Set (T)"=FALSE, "Reference n"=w277, "AlliGator IV DVR in"=w282) -> ("error out"=w279:errorcluster, "[Phasor Plot(s) locked to Ref n"=w280:i32[], "AlliGator IV DVR out"=w281:refnum<data-value>)  [unwired: 6 in]
      n85 = expression code="pi/2-x"(w297) -> (w296:dbl)
      n86 = call "AlliGator Update Phasor References v2.vi"("XYGraph in"=w286, "Phasor Frequency"=w295, "Phase Lifetime 1"=w284, "Phase Lifetime 2"=w283, "New Reference Phase"=w296, "Error In"=w279, "Locked Plots"=w280, "Updated Reference ID"=w277) -> ("Reference Phasor 1"=w293:T26, "Reference Lifetime 1"=w292:dbl[unit], "Reference Phasor 2"=w291:T26, "Reference Lifetime 2"=w290:dbl[unit], "Error Out"=w289:errorcluster)  [unwired: 3 in]
      n87 = call "AlliGator Get-Set Phasor Ratio References.vi"("Reference Phasor 1"=w293, "Reference Lifetime 1"=w292, "Reference Phasor 2"=w291, "Reference Lifetime 2"=w290, "error in (no error)"=w289, "Get(F)/Set"=TRUE) -> ("error out"=w288:errorcluster)  [unwired: 2 in, 7 out]
    }
    frame "Phasor Ratio:Update Phasor Reference 2" {
      w301 = 2 ("Updated Reference ID")
      # "\"Update Phasor Reference 2\""
      n88 = call-poly "Variant to Data.vi"("Variant"=w320) -> ("Value"=w319:dbl)  [unwired: 8 in]
      n89 = Unbundle By Name(w307) -> ("Registered Events Ctrl Refnums.Phasor Graph"=w308:refnum<vi>, "Phasor Graph Ctrl Refnums.Phase Lifetime 1"=w306:refnum<vi>, "Phasor Graph Ctrl Refnums.Phase Lifetime 2"=w305:refnum<vi>)
      n90 = call "AlliGator IV Phasor Plots Locked to Reference n.vi"("Get (F)/ Set (T)"=FALSE, "Reference n"=w301, "AlliGator IV DVR in"=w304) -> ("error out"=w299:errorcluster, "[Phasor Plot(s) locked to Ref n"=w302:i32[], "AlliGator IV DVR out"=w303:refnum<data-value>)  [unwired: 6 in]
      n91 = expression code="pi/2-x"(w319) -> (w318:dbl)
      n92 = call "AlliGator Update Phasor References v2.vi"("XYGraph in"=w308, "Phasor Frequency"=w317, "Phase Lifetime 1"=w306, "Phase Lifetime 2"=w305, "New Reference Phase"=w318, "Error In"=w299, "Locked Plots"=w302, "Updated Reference ID"=w301) -> ("Reference Phasor 1"=w315:T26, "Reference Lifetime 1"=w314:dbl[unit], "Reference Phasor 2"=w313:T26, "Reference Lifetime 2"=w312:dbl[unit], "Error Out"=w311:errorcluster)  [unwired: 3 in]
      n93 = call "AlliGator Get-Set Phasor Ratio References.vi"("Reference Phasor 1"=w315, "Reference Lifetime 1"=w314, "Reference Phasor 2"=w313, "Reference Lifetime 2"=w312, "error in (no error)"=w311, "Get(F)/Set"=TRUE) -> ("error out"=w310:errorcluster)  [unwired: 2 in, 7 out]
    }
    frame "Phasor Ratio:Use as Phasor Reference 1 Lifetime" {
      w323 = TRUE ("Set (T)/Unset (F)")
      # "\"Use as Phasor Reference 1 Lifetime\""
      n94 = Unbundle By Name(w327) -> ("Other AlliGator Ctrl Refnums.State Indicators"=w326:refnum<vi>)
      n95 = call "AlliGator Build Reference Lifetime String.vi"("Reference #"=1, "Lifetime"=w328) -> ("Error Out"=w332:errorcluster, "Message"=w324:string)  [unwired: 8 in]
      n96 = call "AlliGator Get-Set State Indicators.vi"("State Indicators Refnum"=w326, "AlliGator State Indicators List"=AlliGator_State_Indicators_List."Lifetime Reference 1 Defined" ("Time-Gated Phasor Analysis Task List"), "Error In"=w332, "ON/OFF"=w323, "Set (T)/Get"=w323) -> ("Error Out"=w331:errorcluster)  [unwired: 8 in, 2 out]
      n97 = call "Alligator Variables Storage.vi"("Get(F)/Set"=w323, "AlliGator Variable"=AlliGator_Variables_List."Phasor Plot:Lifetime Reference 1" ("Alligator Variable"), "Error In"=w331, "Data in"=w328) -> ("Error Out"=w330:errorcluster)  [unwired: 5 in, 2 out]
    }
    frame "Phasor Ratio:Use as Phasor Reference 2 Lifetime" {
      w338 = TRUE ("Set (T)/Unset (F)")
      # "\"Use as Phasor Reference 2 Lifetime\""
      n98 = Unbundle By Name(w341) -> ("Other AlliGator Ctrl Refnums.State Indicators"=w340:refnum<vi>)
      n99 = call "AlliGator Build Reference Lifetime String.vi"("Reference #"=2, "Lifetime"=w342) -> ("Error Out"=w346:errorcluster)  [unwired: 8 in, 1 out]
      n100 = call "AlliGator Get-Set State Indicators.vi"("State Indicators Refnum"=w340, "AlliGator State Indicators List"=AlliGator_State_Indicators_List."Lifetime Reference 2 Defined" ("Time-Gated Phasor Analysis Task List"), "Error In"=w346, "ON/OFF"=w338, "Set (T)/Get"=w338) -> ("Error Out"=w345:errorcluster)  [unwired: 8 in, 2 out]
      n101 = call "Alligator Variables Storage.vi"("Get(F)/Set"=w338, "AlliGator Variable"=AlliGator_Variables_List."Phasor Plot:Lifetime Reference 2" ("Alligator Variable"), "Error In"=w345, "Data in"=w342) -> ("Error Out"=w344:errorcluster)  [unwired: 5 in, 2 out]
    }
    frame "Phasor Ratio:Use as Reference n" {
      # "\"Use as Reference n\""
      n102 = call "AlliGator IV Last Calibrated Phasor.vi"("Get (F)/ Set (T)"=FALSE, "AlliGator IV DVR in"=w359) -> ("error out"=w357:errorcluster, "Last Calibrated Phasor"=w358:T26, "AlliGator IV DVR out"=w355:refnum<data-value>)  [unwired: 7 in]
      n103 = Unbundle By Name(w369) -> ("Other AlliGator Ctrl Refnums.State Indicators"=w371:refnum<vi>, "Registered Events Ctrl Refnums.Phasor Graph"=w379:refnum<vi>, "Phasor Graph Ctrl Refnums"=w370:T11)
      n104 = call "Show Animated Busy Icon with Message.vi"("Already active? (F)"=w354, "Message"=w367, "Error In"=w357, "Target VI Refnum"=w368) -> ("Error Out"=w374:errorcluster)  [unwired: 7 in]
      n105 = Unbundle By Name(w369) -> ("Phasor Graph Ctrl Refnums.Phase Lifetime 1"=w362:refnum<vi>, "Phasor Graph Ctrl Refnums.Phase Lifetime 2"=w361:refnum<vi>)
      n106 = call "AlliGator Get Phasor Ratio Reference v2.vi"("Error In"=w374, "Last Phasor"=w358, "Data"=w381) -> ("error out"=w378:errorcluster, "Reference #"=w365:i32, "Reference Phasor"=w372:T26)  [unwired: 6 in]
      n107 = Decrement(x=w365) -> (x-1=w364:i32)
      n108 = Equal To 0?(x=w364) -> (x = 0?=w363:bool)
      n109 = call "AlliGator Update Phasor Graph Information at Cursor.vi"("Valid?"=TRUE, "Error In"=w378, "Phasor"=w372, "Current Phasor Information Indicators"=w370) -> ("Error Out"=w377:errorcluster, "Phase Lifetime"=w375:dbl[unit])  [unwired: 6 in]
      n110 = Select(t=w362, s=w363, f=w361) -> (s? t:f=w360:refnum<vi>)
      n111 = call "AlliGator Set Phasor Reference.vi"("Lifetime"=w375, "State Indicators Refnum"=w371, "error in (no error)"=w377, "Reference Number"=w365, "Plot Data Point"=w372, "Phasor Graph Refnum"=w379) -> ("Error Out"=w376:errorcluster, "Message"=w352:string)  [unwired: 4 in]
      n112 = property class="DigNum (strict)"(reference=w360, "Value"=w375, "Visible"=TRUE) -> ()  [unwired: 1 in, 2 out]
      n113 = call "Hide Animated Busy Icon with Message.vi"("Already active? (F)"=w354, "Error In"=w376, "Target VI reference"=w368) -> ("Error Out"=w373:errorcluster)  [unwired: 8 in]
    }
  }
  "Data Value Reference out" <- w6
  "error out" <- w16
  "Script out" <- w10
  "AlliGator Q Elements out" <- w9
  n114 = call "Get Current Message Text Format.vi"("Text Format"=w1) -> ("Message Formatting"=w3:T2)  [unwired: 8 in, 1 out]
  n115 = call "AlliGator Package Notebook Messages.vi"("Message Formatting"=w3, "Message"=w5, "AlliGator Q Event in"="AlliGator Q Event in") -> ("[Notebook Message]"=→"[Notebook Message]":T1[])  [unwired: 8 in]
